vi "Vision.vi"(11 "Image In":T3) -> (0 "Angle":sgl, 1 "Distance":dbl, 3 "Image Out":T3)   [LabVIEW 2014]
uses:
  <vilib>/vision/Image Controls.llb/IMAQ Image.ctl
  <vilib>/vision/Pattern Matching.llb/IMAQ GM Match Report.ctl
  <vilib>/vision/Pattern Matching.llb/IMAQ Curve Parameters.ctl
  <vilib>/vision/Pattern Matching.llb/IMAQ Match Range Setting.ctl
  <vilib>/vision/NI_Vision_Development_Module.lvlib
panel:
  out "Calibrated Matches":T1[](array[typedef]) {"Correlation Score" format="%.2f"; "Target Template Curve Score" format="%.2f"; "Template Target Curve Score" format="%.2f"; "Bounding Box"."y" format="%.2f"; "Bounding Box"."x" format="%.2f"; "Position"."y" format="%.2f"; "Position"."x" format="%.2f"; "Score" format="%.2f"; "Scale" format="%.2f"; "Angle" format="%.2f"; "Occlusion %" format="%.2f"}
  out "Results (Calibrated)":sgl[][](array[numeric]) format="%.2f"
  out "Results (Pixels)":sgl[][](array[numeric]) format="%.2f"
  out "Shape Report (calibrated)":T2(array[cluster]) {"Score" format="%.2f"; "Centroid"."y" format="%.2f"; "Centroid"."x" format="%.2f"}
  out "error out":errorcluster
  in  "error in":errorcluster
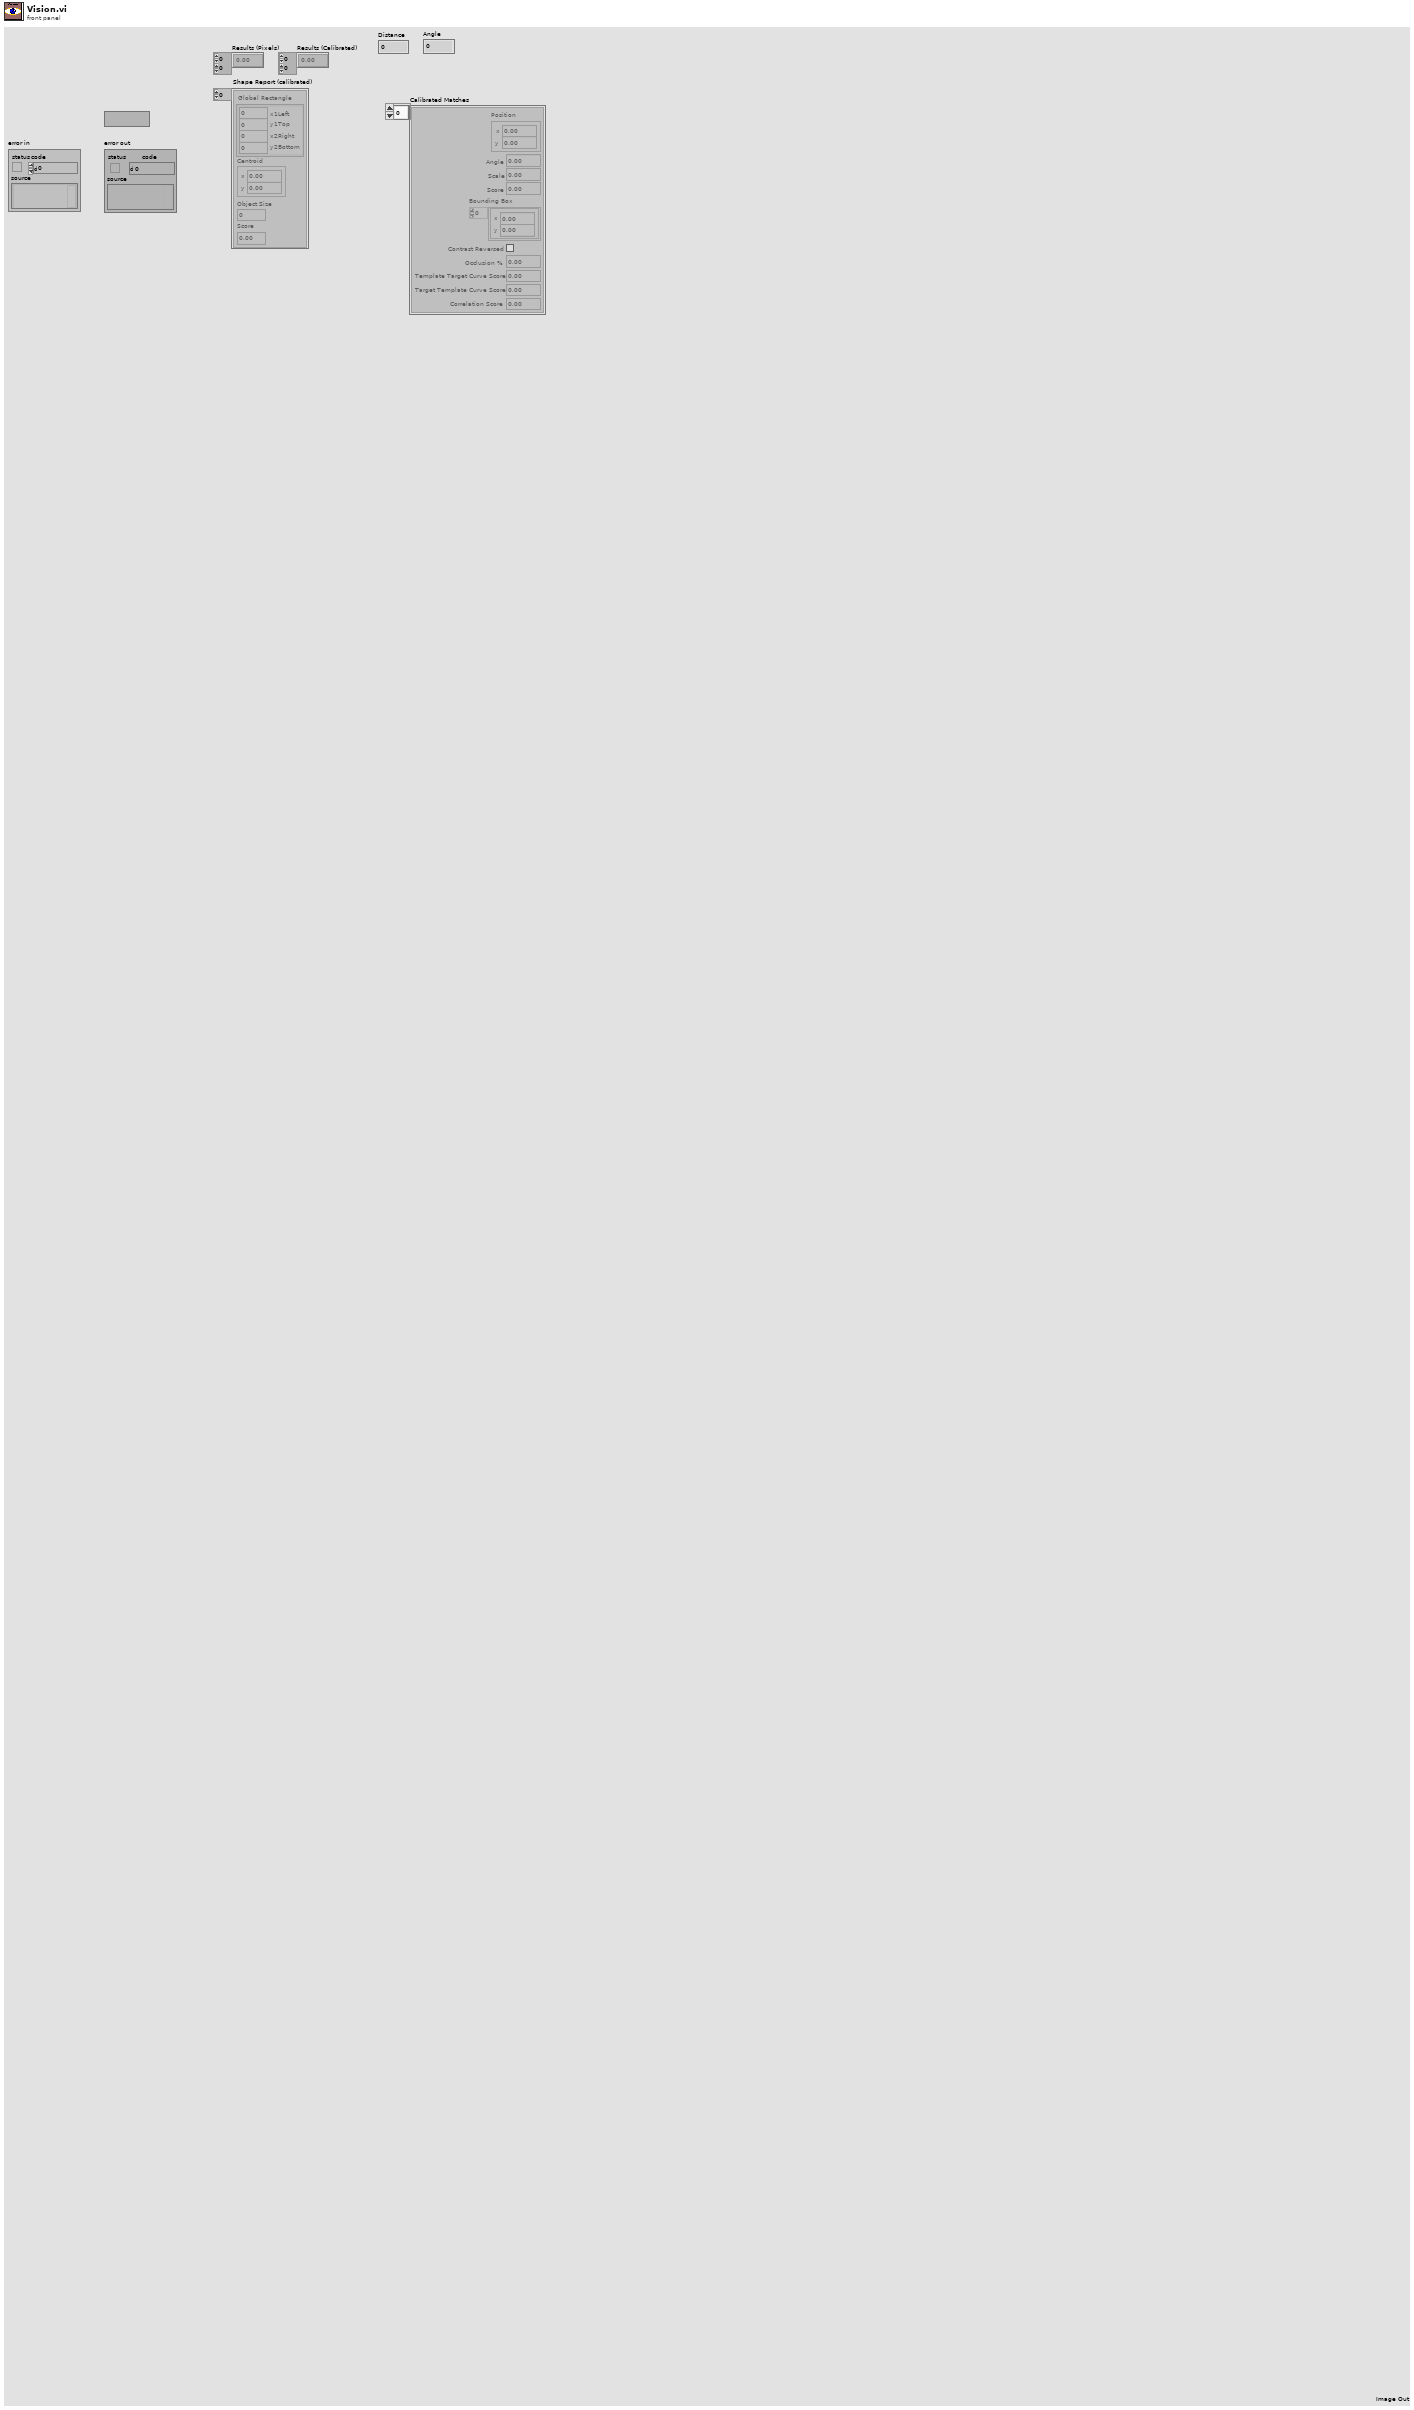
[diagram p1: front panel]
types:
  T1 = typedef "IMAQ GM Match Report.ctl" = cluster{"Position":cluster{"x":sgl, "y":sgl}, "Angle":sgl, "Scale":sgl, "Score":sgl, "Bounding Box":cluster{"x":sgl, "y":sgl}[], "Contrast Reversed":bool, "Occlusion %":sgl, "Template Target Curve Score":sgl, "Target Template Curve Score":sgl, "Correlation Score":sgl}
  T2 = cluster{"Global Rectangle":cluster{"x1Left":i32, "y1Top":i32, "x2Right":i32, "y2Bottom":i32}, "Centroid":cluster{"x":sgl, "y":sgl}, "Object Size":u32, "Score":dbl}[]
  T3 = typedef "IMAQ Image.ctl" = refnum<image>
  T4 = cluster{"Feature":u32, "Points IDs":cluster{"GUID":string, "Index":i32}[]}[]
  T5 = typedef "IMAQ Curve Parameters.ctl" = cluster{"Extraction Mode":u32, "Edge Threshold":i32, "Edge Filter Size":u32, "Min Length":i32, "Row Search Step Size":i32, "Col Search Step Size":i32, "Max Endpoint Gap":i32, "Closed":bool, "Subpixel":bool}
  T6 = typedef "IMAQ Match Range Setting.ctl" = cluster{"Match Constraints":u32, "Min":dbl, "Max":dbl}
  T7 = cluster{"Curve Parameters":T5, "Match Mode":cluster{"Rotation":bool, "Scale":bool, "Occlusion":bool, "Reserved":bool, "Reserved":bool, "Reserved":bool}, "Range Settings":T6[], "Number of Matches":i32, "Minimum Match Score":sgl, "SubPixel Accuracy":bool, "Adv. Geometric Match Options 2":cluster{"Setup Data Item":u16, "Item Value":dbl}[]}
  T8 = cluster{"Global Rectangle":i32[], "Contours":cluster{"ID":enum32{"External", "Internal"}, "Type":u32, "Coordinates":i32[]}[]}
  T9 = enum32{"AutoM", "Close", "Dilate", "Erode", "Gradient", "Gradient in", "Gradient out", "HitMiss", "Open", "PClose", "POpen", "Thick", "Thin"}
  T10 = cluster{"histogram":u32[], "Minimal Value":sgl, "Maximal Value":sgl, "Starting Value":sgl, "Interval Width":sgl, "Mean Value":sgl, "Standard  Variation":sgl, "Area (pixels)":i32}
  T11 = typedef "Image Type" = u32
  T12 = cluster{"Shape Report (calibrated)[0]":cluster{"Global Rectangle":cluster{"x1Left":i32, "y1Top":i32, "x2Right":i32, "y2Bottom":i32}, "Centroid":cluster{"x":sgl, "y":sgl}, "Object Size":u32, "Score":dbl}, "Shape Report (calibrated)[1]":cluster{"Global Rectangle":cluster{"x1Left":i32, "y1Top":i32, "x2Right":i32, "y2Bottom":i32}, "Centroid":cluster{"x":sgl, "y":sgl}, "Object Size":u32, "Score":dbl}, "Shape Report (calibrated)[2]":cluster{"Global Rectangle":cluster{"x1Left":i32, "y1Top":i32, "x2Right":i32, "y2Bottom":i32}, "Centroid":cluster{"x":sgl, "y":sgl}, "Object Size":u32, "Score":dbl}, "Shape Report (calibrated)[3]":cluster{"Global Rectangle":cluster{"x1Left":i32, "y1Top":i32, "x2Right":i32, "y2Bottom":i32}, "Centroid":cluster{"x":sgl, "y":sgl}, "Object Size":u32, "Score":dbl}, "Shape Report (calibrated)[4]":cluster{"Global Rectangle":cluster{"x1Left":i32, "y1Top":i32, "x2Right":i32, "y2Bottom":i32}, "Centroid":cluster{"x":sgl, "y":sgl}, "Object Size":u32, "Score":dbl}, "Shape Report (calibrated)[5]":cluster{"Global Rectangle":cluster{"x1Left":i32, "y1Top":i32, "x2Right":i32, "y2Bottom":i32}, "Centroid":cluster{"x":sgl, "y":sgl}, "Object Size":u32, "Score":dbl}, "Shape Report (calibrated)[6]":cluster{"Global Rectangle":cluster{"x1Left":i32, "y1Top":i32, "x2Right":i32, "y2Bottom":i32}, "Centroid":cluster{"x":sgl, "y":sgl}, "Object Size":u32, "Score":dbl}, "Shape Report (calibrated)[7]":cluster{"Global Rectangle":cluster{"x1Left":i32, "y1Top":i32, "x2Right":i32, "y2Bottom":i32}, "Centroid":cluster{"x":sgl, "y":sgl}, "Object Size":u32, "Score":dbl}, "Shape Report (calibrated)[8]":cluster{"Global Rectangle":cluster{"x1Left":i32, "y1Top":i32, "x2Right":i32, "y2Bottom":i32}, "Centroid":cluster{"x":sgl, "y":sgl}, "Object Size":u32, "Score":dbl}}
  T13 = cluster{"Global Rectangle":cluster{"x1Left":i32, "y1Top":i32, "x2Right":i32, "y2Bottom":i32}, "Centroid":cluster{"x":sgl, "y":sgl}, "Object Size":u32, "Score":dbl}
  T14 = cluster{"Results (Pixels)[0]":sgl, "Results (Pixels)[1]":sgl, "Results (Pixels)[2]":sgl, "Results (Pixels)[3]":sgl, "Results (Pixels)[4]":sgl, "Results (Pixels)[5]":sgl, "Results (Pixels)[6]":sgl, "Results (Pixels)[7]":sgl, "Results (Pixels)[8]":sgl}
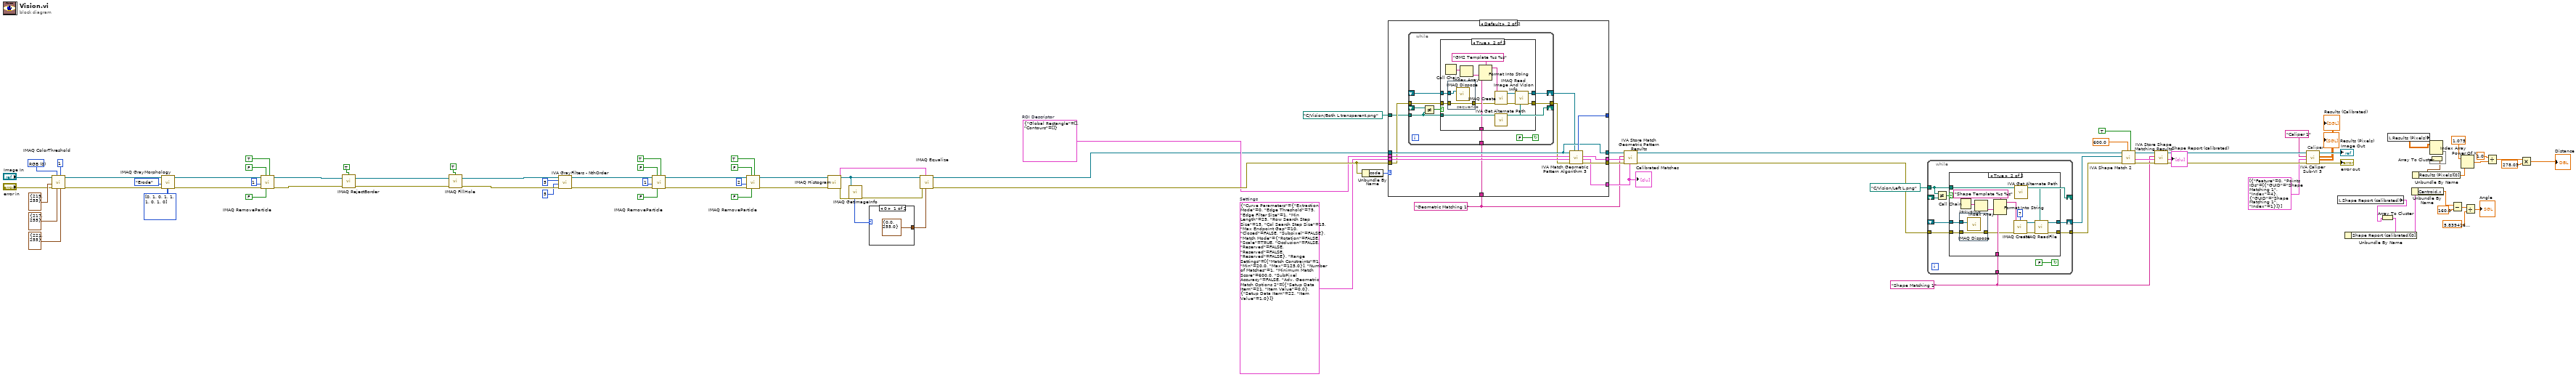
[diagram p0: block diagram]
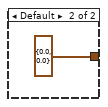
[diagram p5: hidden frame]
diagram:
  w27 = "Shape Matching 1" ("Step Name")
  w39 = T7 {"Curve Parameters"={"Extraction Mode"=0, "Edge Threshold"=75, "Edge Filter Size"=1, "Min Length"=25, "Row Search Step Size"=15, "Col Search Step Size"=15, "Max Endpoint Gap"=10, "Closed"=FALSE, "Subpixel"=FALSE}, "Match Mode"={"Rotation"=FALSE, "Scale"=TRUE, "Occlusion"=FALSE, "Reserved"=FALSE, "Reserved"=FALSE, "Reserved"=FALSE}, "Range Settings"=[{"Match Constraints"=1, "Min"=20.0, "Max"=125.0}], "Number of Matches"=1, "Minimum Match Score"=600.0, "SubPixel Accuracy"=FALSE, "Adv. Geometric Match Options 2"=[{"Setup Data Item"=21, "Item Value"=0.0}, {"Setup Data Item"=22, "Item Value"=1.0}]}  # Settings
  w38 = "Geometric Matching 1" ("Step Name")
  w47 = T8 {"Global Rectangle"=[], "Contours"=[]}  # ROI Descriptor
  w94 = u16 0 items=["RGB", "HSL", "HSV", "HSI"] ("Color Mode")
  # "Caliper"
  n1 = call "IMAQ ColorThreshold"("Blue or Luma or Val or Inten Range"=cluster{"Lower value":i32, "Upper value":i32} {"Lower value"=221, "Upper value"=255}, "Replace Value"=1, "Green or Sat Range"=cluster{"Lower value":i32, "Upper value":i32} {"Lower value"=217, "Upper value"=255}, "Color Mode"=w94, "error in (no error)"="error in", "Red or Hue Range"=cluster{"Lower value":i32, "Upper value":i32} {"Lower value"=219, "Upper value"=255}, "Image Src"="Image In") -> ("error out"=w88:errorcluster, "Image Dst Out"=w85:T3)  [unwired: 1 in, 2 out]
  n2 = call "IMAQ GrayMorphology"("Structuring Element"=i32[][] [[0, 1, 0], [1, 1, 1], [0, 1, 0]], "error in (no error)"=w88, "Operation"=T9."Erode", "Image Src"=w85) -> ("error out"=w84:errorcluster, "Image Dst Out"=w79:T3)  [unwired: 3 in, 3 out]
  n3 = call "IMAQ RemoveParticle"("Connectivity 4/8 (8)"=TRUE, "Low Pass/High Pass (Low)"=FALSE, "Square/Hexa (Square)"=FALSE, "error in (no error)"=w84, "Number of Erosion"=1, "Image Src"=w79) -> ("error out"=w78:errorcluster, "Image Dst Out"=w76:T3)  [unwired: 1 in, 3 out]
  n4 = call "IMAQ RejectBorder"("error in (no error)"=w78, "Image Src"=w76, "Connectivity 4/8 (8)"=TRUE) -> ("error out"=w75:errorcluster, "Image Dst Out"=w73:T3)  [unwired: 1 in, 2 out]
  n5 = call "IMAQ FillHole"("error in (no error)"=w75, "Image Src"=w73, "Connectivity 4/8 (8)"=TRUE) -> ("error out"=w72:errorcluster, "Image Dst Out"=w71:T3)  [unwired: 1 in, 2 out]
  n6 = call <vilib>:"IVA GrayFilters - NthOrder.vi"("error in"=w72, "Filter size Y"=5, "Filter size X"=5, "Image In"=w71) -> ("error out"=w70:errorcluster, "Image Out"=w63:T3)  [unwired: 6 out]
  n7 = call "IMAQ RemoveParticle"("Connectivity 4/8 (8)"=TRUE, "Low Pass/High Pass (Low)"=FALSE, "Square/Hexa (Square)"=FALSE, "error in (no error)"=w70, "Number of Erosion"=1, "Image Src"=w63) -> ("error out"=w62:errorcluster, "Image Dst Out"=w57:T3)  [unwired: 1 in, 3 out]
  n8 = call "IMAQ RemoveParticle"("Connectivity 4/8 (8)"=TRUE, "Low Pass/High Pass (Low)"=FALSE, "Square/Hexa (Square)"=FALSE, "error in (no error)"=w62, "Number of Erosion"=2, "Image Src"=w57) -> ("error out"=w56:errorcluster, "Image Dst Out"=w52:T3)  [unwired: 1 in, 3 out]
  n9 = call "IMAQ Histogram"("error in (no error)"=w56, "Image"=w52) -> ("error out"=w51:errorcluster, "Histogram Report"=w54:T10)  [unwired: 3 in, 5 out]
  n10 = call "IMAQ GetImageInfo"("error in (no error)"=w51, "Image"=w52) -> ("error out"=w50:errorcluster, "Image Type"=w53:T11)  [unwired: 8 out]
  n11 = case shown="0" w53 {
    tunnel: [cluster{"Minimum":sgl, "Maximum":sgl} {"Minimum"=0.0, "Maximum"=255.0} ("Range") cluster{"Minimum":sgl, "Maximum":sgl} {"Minimum"=0.0, "Maximum"=0.0} ("Range")] -> w49
    frame 0 {
    }
    frame Default {
    }
  }
  n12 = call "IMAQ Equalize"("Range"=w49, "Histogram Report"=w54, "error in (no error)"=w50, "Image Src"=w52) -> ("error out"=w55:errorcluster, "Image Dst Out"=w46:T3)  [unwired: 2 in, 4 out]
  n13 = Unbundle By Name(w55) -> ("code"=w41:i32)
  n14 = case shown="Default" w41 {
    tunnel: path "C:/Vision/Both L transparent.png" ("Template File Path") -> [_ w100]
    tunnel: w55 -> [_ w101]
    tunnel: w39 -> [_ w110]
    tunnel: w47 -> [_ w109]
    tunnel: w46 -> [w98 w104]
    tunnel: [_ w108] -> w45
    tunnel: [_ w107] -> w43
    tunnel: [_ w106] -> w42
    tunnel: [_ w105] -> _
    tunnel: [w98 w104] -> w40
    tunnel: w38 -> [_ w99]
    frame -1074396199, -1074396198 {
      # "Discard Coordinate System Error"
    }
    frame Default {
      n15 = while {
        shift-right: [w119] -> w102
        shift-left: _ -> [w118]
        tunnel: [w116] -> w103
        tunnel: w101 -> [w115]
        tunnel: w100 -> [w111]
        tunnel: w99 -> [w114]
        shift-right: [w111] -> _
        shift-left: _ -> [w113]
        stop <- FALSE continue-if-true
        n16 = Not Equal?(x=w113, y=w111) -> (x != y?=w112:bool)
        n17 = case shown="True" w112 {
          tunnel: [w121 w133] -> w119
          tunnel: w118 -> [w121 w125]
          tunnel: [w120 w130] -> w116
          tunnel: w115 -> [w120 w126]
          tunnel: w114 -> [_ w127]
          tunnel: w111 -> [_ w123]
          frame False {
          }
          frame True {
            n18 = Call Chain() -> (call chain=w129:string[])
            n19 = stacked-sequence {
              tunnel: w126 -> [w137]
              tunnel: w125 -> [w136]
              tunnel: [w137] -> w124
              frame #0 {
                n20 = call "IMAQ Dispose"("Image"=w136) -> ()  [unwired: 2 in, 4 out]
              }
            }
            n21 = Index Array(array=w129) -> (element=w128:string)  [unwired: 1 in]
            n22 = Format Into String(format string="GM2 Template %s %s" ("Image Name"), w128, w127) -> (resulting string=w135:string)  [unwired: 2 in, 1 out]
            n23 = call "IMAQ Create"("Image Name"=w135, "error in (no error)"=w124) -> ("New Image"=w132:T3, "error out"=w131:errorcluster)  [unwired: 2 in, 1 out]
            n24 = call <vilib>:"IVA Get Alternate Path.vi"("Path In"=w123) -> ("Path Out"=w122:path)  [unwired: 10 out]
            n25 = call "IMAQ Read Image And Vision Info"("File Path"=w122, "error in (no error)"=w131, "Image"=w132) -> ("error out"=w130:errorcluster, "Image Out"=w133:T3)  [unwired: 1 in, 6 out]
          }
        }
      }
      n26 = call <vilib>:"IVA Match Geometric Pattern Algorithm 3.vi"("Template"=w102, "error in (no error)"=w103, "Settings"=w110, "ROI Descriptor"=w109, "Image"=w104) -> ("error out"=w108:errorcluster, "Calibrated Matches"=w106:T1[], "Matches"=w107:T1[], "Number of Matches"=w105:i32)  [unwired: 3 out]
    }
  }
  "Calibrated Matches" <- w42
  n27 = call <vilib>:"IVA Store Match Geometric Pattern Results.vi"("Calibrated Matches"=w42, "error in (no error)"=w45, "Matches"=w43, "Step Name"=w38, "Image in"=w40) -> ("error out"=w44:errorcluster, "Image dup"=w35:T3)  [unwired: 5 out]
  n28 = while {
    shift-right: [w146] -> w28
    shift-left: _ -> [w145]
    tunnel: [w143] -> w29
    tunnel: w44 -> [w142]
    tunnel: path "C:/Vision/Left L.png" ("Template Path") -> [w140]
    tunnel: w27 -> [w141]
    shift-right: [w140] -> _
    shift-left: _ -> [w139]
    stop <- FALSE continue-if-true
    n29 = Not Equal?(x=w140, y=w139) -> (x != y?=w138:bool)
    n30 = case shown="True" w138 {
      tunnel: [w148 w160] -> w146
      tunnel: w145 -> [w148 w151]
      tunnel: [w147 w158] -> w143
      tunnel: w142 -> [w147 w150]
      tunnel: w140 -> [_ w153]
      tunnel: w141 -> [_ w154]
      frame False {
      }
      frame True {
        n31 = Call Chain() -> (call chain=w156:string[])
        n32 = stacked-sequence {
          tunnel: w151 -> [w165]
          tunnel: w150 -> [w164]
          tunnel: [w164] -> w149
          frame #0 {
            n33 = call "IMAQ Dispose"("Image"=w165) -> ()  [unwired: 2 in, 4 out]
          }
        }
        n34 = Index Array(array=w156) -> (element=w155:string)  [unwired: 1 in]
        n35 = Format Into String(format string="Shape Template %s %s" ("Image Name"), w155, w154) -> (resulting string=w163:string)  [unwired: 2 in, 1 out]
        n36 = call "IMAQ Create"("Border Size"=7, "Image Name"=w163, "error in (no error)"=w149) -> ("New Image"=w161:T3, "error out"=w159:errorcluster)  [unwired: 1 in, 1 out]
        n37 = call <vilib>:"IVA Get Alternate Path.vi"("Path In"=w153) -> ("Path Out"=w152:path)  [unwired: 10 out]
        n38 = call "IMAQ ReadFile"("File Path"=w152, "error in (no error)"=w159, "Image"=w161) -> ("error out"=w158:errorcluster, "Image Out"=w160:T3)  [unwired: 2 in, 5 out]
      }
    }
  }
  n39 = call <vilib>:"IVA Shape Match 2.vi"("Scale Invariance"=TRUE, "Minimal Score"=600.0, "error in (no error)"=w29, "Template"=w28, "Image Src"=w35) -> ("error out"=w34:errorcluster, "Shape Report"=w32:T2, "Image Out"=w31:T3)  [unwired: 4 out]
  n40 = call <vilib>:"IVA Store Shape Matching Results.vi"("error in (no error)"=w34, "Shape Report"=w32, "Step Name"=w27, "Image in"=w31) -> ("error out"=w33:errorcluster, "Shape Report (calibrated)"=→"Shape Report (calibrated)":T2, "Image dup"=w26:T3)  [unwired: 5 out]
  n41 = call <vilib>:"IVA Caliper Sub-VI 3.vi"("error in"=w33, "Parameters"=T4 [{"Feature"=0, "Points IDs"=[{"GUID"="Shape Matching 1", "Index"=4}, {"GUID"="Shape Matching 1", "Index"=1}]}], "Step Name"="Caliper 1", "Image In"=w26) -> ("error out"=→"error out":errorcluster, "Results (Calibrated)"=→"Results (Calibrated)":sgl[][], "Results (Pixels)"=→"Results (Pixels)":sgl[][], "Image Out"=→"Image Out":T3)  [unwired: 1 in, 3 out]
  n42 = local read "Shape Report (calibrated)"() -> (w4:T2)
  n43 = Array To Cluster(array=w4) -> (cluster=w3:T12)
  n44 = Unbundle By Name(w3) -> ("Shape Report (calibrated)[0]"=w2:T13)
  n45 = local read "Results (Pixels)"() -> (w9:sgl[][])
  n46 = Unbundle By Name(w2) -> ("Centroid.x"=w18:sgl)
  n47 = Index Array(array=w9) -> (element=w8:sgl[])  [unwired: 2 in]
  n48 = Array To Cluster(array=w8) -> (cluster=w7:T14)
  n49 = Unbundle By Name(w7) -> ("Results (Pixels)[0]"=w6:sgl)
  n50 = Subtract(x=w18, y=sgl 160.0) -> (x-y=w16:sgl)
  n51 = Power Of X(1:w6, 2:1.075 ("x")) -> (0:w12:dbl)
  n52 = Divide(x=w16, y=sgl 5.839416) -> (x/y=→"Angle":sgl)
  n53 = Divide(x=1.0, y=w12) -> (x/y=w11:dbl)
  n54 = Multiply(x=w11, y=278.03) -> (x*y=→"Distance":dbl)
